vi "Thermal Chamber Controller.vi"   [LabVIEW 2015]
doc: "Implements a Thermal Chamber Controller with a <b>singleton</b> Delacor QMH module. The chamber is configured to reach a temperature set point. Once the temperature is reached the VI stops.\n\nThis example illustrates that there is no need to have an event structure in the calling code and provides an example of a traditional \"Configure > Read/Write > Close\" application.\n____\nDelacor QMH Thermal Chamber Examples 4.0.0.21\nCopyright (c) 2018, Delacor"
uses:
  Libraries/Thermal Chamber Controller_DQMH/Heater State--enum.ctl
  Libraries/Thermal Chamber Controller_DQMH/Thermal Chamber Controller_DQMH.lvlib
panel:
  # "Overview: Demonstrates how to implement a Thermal Chamber Controller with a singleton Delacor QMH Module.\nRequirements: Delacor QMH\nInstructions:\n1. Run the VI to launch the singleton Thermal Chamber Controller DQMH module.\n2. Observe the temperature in the Thermal Chamber rise as it approaches the set point.\n3. Once the set point is reached, the example will stop. See the block diagram of this VI for more information."
types:
  T1 = typedef "Thermal Chamber Controller_DQMH.lvlib/Heater State--enum.ctl" = enum16{"Heater Enabled", "Heater Disabled"}
  T2 = typedef "Thermal Chamber Controller_DQMH.lvlib/Request and Wait for Status (Reply Payload)--cluster.ctl" = cluster{"Actual Temperature":dbl, "Temperature Set Point":dbl, "Temperature Ramp Rate":dbl, "Heater State":T1, "error":errorcluster}
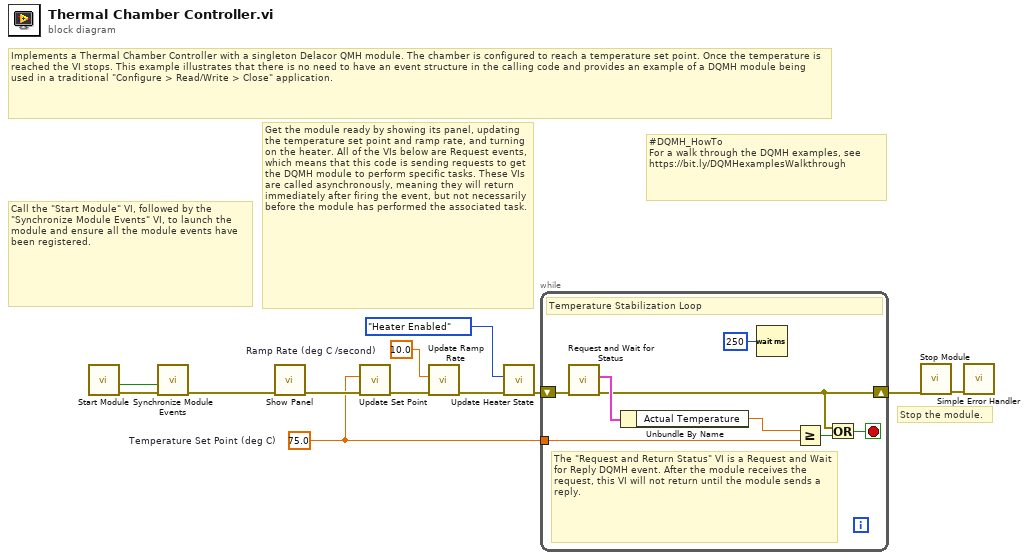
[diagram p0: block diagram]
diagram:
  w3 = 10.0  # Ramp Rate (deg C /second)
  w2 = 75.0  # Temperature Set Point (deg C)
  # "#DQMH_HowTo \nFor a walk through the DQMH examples, see https://bit.ly/DQMHexamplesWalkthrough"
  # "Get the module ready by showing its panel, updating the temperature set point and ramp rate, and turning on the heater. All of the VIs below are Request events, which means that this code is sending requests to get the DQMH module to perform specific tasks. These VIs are called asynchronously, meaning they will return immediately after firing the event, but not necessarily before the module has performed the associated task."
  # "Call the \"Start Module\" VI, followed by the \"Synchronize Module Events\" VI, to launch the module and ensure all the module events have been registered."
  # "Implements a Thermal Chamber Controller with a singleton Delacor QMH module. The chamber is configured to reach a temperature set point. Once the temperature is reached the VI stops. This example illustrates that there is no need to have an event structure in the calling code and provides an example of a DQMH module being used in a traditional \"Configure > Read/Write > Close\" application."
  # "Stop the module."
  n1 = call "Start Module.vi"() -> ("error out"=w7:errorcluster, "Wait for Event Sync?"=w4:bool)  [unwired: 8 in, 2 out]
  n2 = call "Synchronize Module Events.vi"("error in (no error)"=w7, "Wait for Event Sync?"=w4) -> ("error out"=w6:errorcluster)  [unwired: 9 in]
  n3 = call "Show Panel.vi"("error in (no error)"=w6) -> ("error out"=w5:errorcluster)  [unwired: 10 in]
  n4 = call "Update Set Point.vi"("error in (no error)"=w5, "Temperature Set Point"=w2) -> ("error out"=w9:errorcluster)  [unwired: 9 in]
  n5 = call "Update Ramp Rate.vi"("error in (no error)"=w9, "Temperature Ramp Rate"=w3) -> ("error out"=w8:errorcluster)  [unwired: 9 in]
  n6 = call "Update Heater State.vi"("error in (no error)"=w8, "Heater State"=Heater_State--enum."Heater Enabled") -> ("error out"=w12:errorcluster)  [unwired: 9 in]
  n7 = while {
    shift-right: [w13] -> w11
    shift-left: w12 -> [w17]
    tunnel: w2 -> [w20]
    stop <- w14 stop-if-true
    # "The \"Request and Return Status\" VI is a Request and Wait for Reply DQMH event. After the module receives the request, this VI will not return until the module sends a reply."
    # "Temperature Stabilization Loop"
    n8 = call "Request and Wait for Status.vi"("error in (no error)"=w17) -> ("error out"=w13:errorcluster, "Reply Payload"=w16:T2)  [unwired: 8 in, 1 out]
    n9 = Unbundle By Name(w16) -> ("Actual Temperature"=w18:dbl)
    n10 = Wait (ms)(milliseconds to wait=u32 250) -> ()  [unwired: 1 out]
    n11 = Greater Or Equal?(x=w18, y=w20) -> (x >= y?=w19:bool)
    n12 = Or(x=w13, y=w19) -> (x .or. y?=w14:bool)
  }
  n13 = call "Stop Module.vi"("error in (no error)"=w11) -> ("error out"=w10:errorcluster)  [unwired: 10 in]
  n14 = call <vilib>:"Simple Error Handler.vi"("error in (no error)"=w10) -> ()  [unwired: 4 in, 5 out]
